vi "Do.vi"(8 "error in (no error)":errorcluster, 10 "Actor in":refnum<class "Actor.lvclass">, 11 "Unregister Edit Test Channel Sensor Names Msg in":refnum<class "Unregister Edit Test Channel Sensor Names Msg.lvclass">) -> (0 "error out":errorcluster, 2 "Actor out":refnum<class "Actor.lvclass">)   [LabVIEW 2013, in "Edit Test Channel Model.lvlib" / "Unregister Edit Test Channel Sensor Names Msg.lvclass"]
doc: "(<B>Filename</B>: Actor Framework.lvlib:Message.lvclass:Do.vi)\n\nDefines what a message does when it is received by an actor. Generally, a message instructs an actor to invoke one of its methods.\n\nBy default, this method does nothing. A child class must override it to define behavior. Create a child class by using the Actor Framework Message Maker dialog box."
uses:
  Unregister Edit Test Channel Sensor Names Msg.lvclass
  <vilib>/ActorFramework/Actor/Actor.lvclass
  Edit Test Channel Model/Edit Test Channel Model.lvclass
  <vilib>/ActorFrameworkMVC/View Observer/Unregistration Message/Unregistration Message.lvclass/Unregistration Message.ctl
  <vilib>/ActorFramework/Message Enqueuer/Message Enqueuer.lvclass
  <vilib>/ActorFrameworkMVC/View Observer/Unregistration Message/Unregistration Message.lvclass
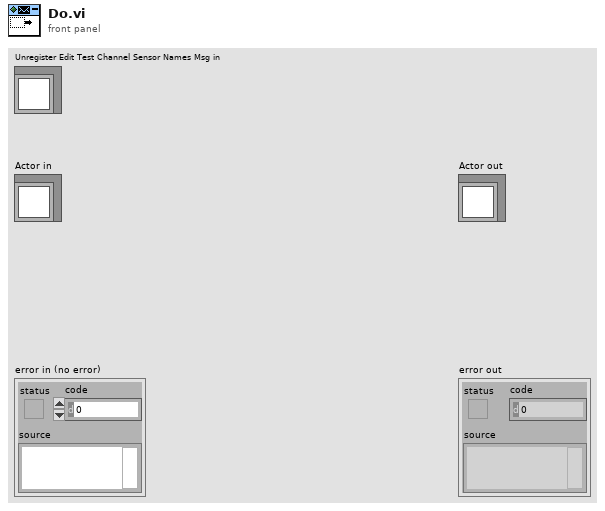
[diagram p1: front panel]
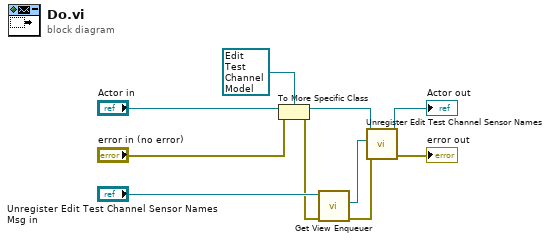
[diagram p0: block diagram]
diagram:
  n1 = To More Specific Class(target class=refnum<class "Edit Test Channel Model.lvclass"> refnum ("Edit Test Channel Model.lvlib:Edit Test Channel Model.lvclass"), reference="Actor in", error in="error in (no error)") -> (specific class reference=w1:refnum<class "Edit Test Channel Model.lvclass">, error out=w4:errorcluster)
  n2 = call <vilib>:"Get View Enqueuer.vi"("error in (no error)"=w4, "Unregistration Message in"="Unregister Edit Test Channel Sensor Names Msg in") -> ("error out"=w2:errorcluster, "View Enqueuer"=w6:refnum<class "Message Enqueuer.lvclass">)  [unwired: 7 in, 1 out]
  n3 = call "Unregister Edit Test Channel Sensor Names.vi"("error in (no error)"=w2, "View Enqueuer"=w6, "Edit Test Channel Model in"=w1) -> ("error out"=→"error out":errorcluster, "Edit Test Channel Model out"=→"Actor out":refnum<class "Edit Test Channel Model.lvclass">)  [unwired: 7 in]
